vi "image evaluation function.vi"(3 "output control":T1, 4 "data":variant, 5 "X":dbl[](array[numeric])) -> (0 "error out":errorcluster, 1 "gradient":dbl[](array[numeric]), 2 "f(X)":dbl)   [LabVIEW 2024]
doc: "Use this template VI as a starting point to create an objective function you want to pass to the Unconstrained Optimization VI."
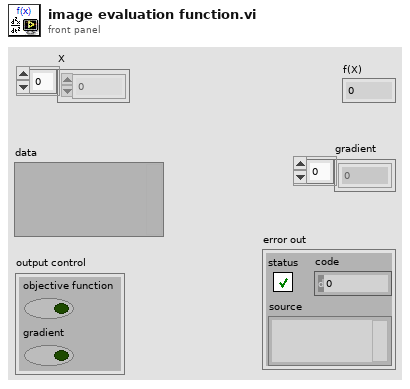
[diagram p1: front panel]
types:
  T1 = cluster{"objective function":bool, "gradient":bool}
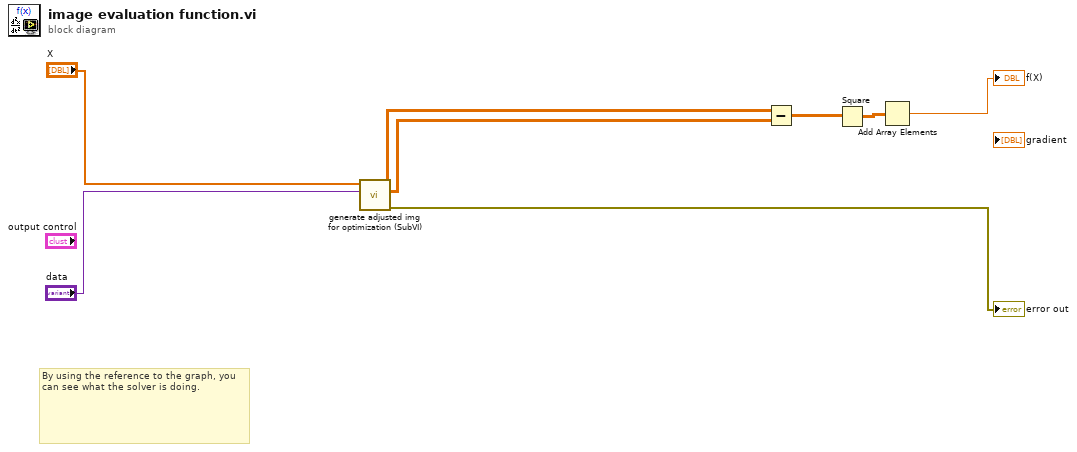
[diagram p0: block diagram]
diagram:
  # "By using the reference to the graph, you can see what the solver is doing."
  n1 = call "generate adjusted img for optimization (SubVI).vi"("data"="data", "X"="X") -> ("error out"=→"error out":errorcluster, "Array"=w6:dbl[][], "GT"=w3:dbl[][])  [unwired: 7 in]
  n2 = Subtract(x=w3, y=w6) -> (x-y=w7:dbl[][])
  n3 = Square(x=w7) -> (x^2=w5:dbl[][])
  n4 = Add Array Elements(numeric array=w5) -> (sum=→"f(X)":dbl)
